vi "Get All Environment Variables [Array of clusters].vi"(7 "Target (Process)":T1 items=["Process", "User", "Machine"], 8 "Error In":errorcluster) -> (0 "Error Out":errorcluster, 3 "Variables[]":T2[](array[typedef]))   [LabVIEW 2023, in "SLL Environment Variable.lvlib"]
doc: "Retrieve all environment variables and their values from the target environment in an array of clusters."
uses:
  SLL Environment Variable.lvlib
  _Typedef/Environment Variable Cluster.ctl
  _Typedef/Target Environment Enum.ctl
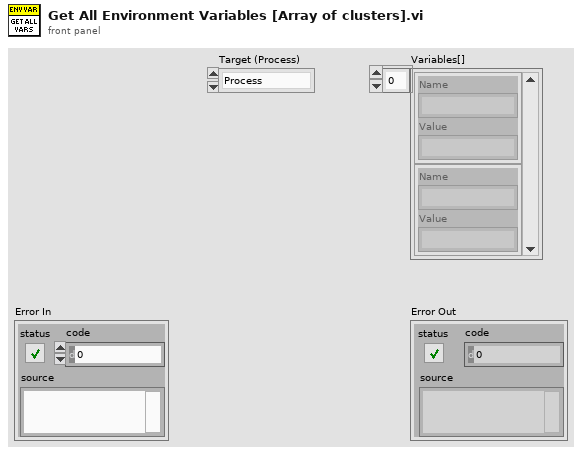
[diagram p1: front panel]
types:
  T1 = typedef "SLL Environment Variable.lvlib/Target Environment Enum.ctl" = i32
  T2 = typedef "SLL Environment Variable.lvlib/Environment Variable Cluster.ctl" = cluster{"Name":string, "Value":string}
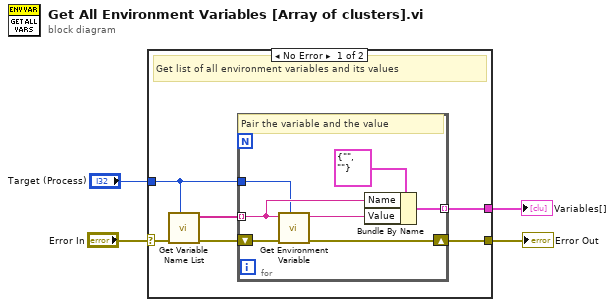
[diagram p0: block diagram]
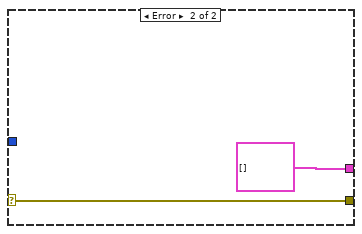
[diagram p2: hidden frame]
diagram:
  n1 = case shown="No Error" "Error In" {
    selector: "Error In" -> [w10 w19]
    tunnel: [w8 w19] -> w4
    tunnel: [w6 T2[] []] -> w3
    tunnel: "Target (Process)" -> [w5 _]
    frame No Error {
      # "Get list of all environment variables and its values"
      n2 = call "Get Variable Name List.vi"("Target (Process)"=w5, "Error In"=w10) -> ("Error Out"=w9:errorcluster, "Names[]"=w7:string[])  [unwired: 8 in]
      n3 = for {
        shift-right: [w16] -> w8
        shift-left: w9 -> [w17]
        tunnel: w7 -> [w15] mode=indexing
        tunnel: [w12] -> w6 mode=indexing
        tunnel: w5 -> [w11]
        # "Pair the variable and the value"
        n4 = call "Get Environment Variable.vi"("Target (Process)"=w11, "Error In"=w17, "Name"=w15) -> ("Error Out"=w16:errorcluster, "Value"=w14:string)  [unwired: 7 in]
        n5 = Bundle By Name(cluster=T2 {"Name"="", "Value"=""}, "Name"=w15, "Value"=w14) -> (w12:T2)
      }
    }
    frame Error {
    }
  }
  "Error Out" <- w4
  "Variables[]" <- w3
